vi "MM2KManCTRL.VI"(0 "MM System":u16(ring)=1 items=["MM3000", "MM2000"]) -> ()   [LabVIEW 2022 SP3]
uses:
  -MotionRoutines/MotionGlobals.vi
panel:
  in  "ExitSendCmd":bool
  out "Ax3Disp":dbl format="%.3f"
  out "Ax2Disp":dbl format="%.3f"
  in  "FineMi3":bool
  in  "FinePl3":bool
  in  "FineMi2":bool
  in  "FinePl2":bool
  in  "FineMi1":bool
  in  "FinePl1":bool
  in  "Rst3":bool
  in  "Ax3Plus":bool
  in  "Ax3Minus":bool
  in  "Rst2":bool
  in  "Ax2Plus":bool
  in  "Ax2Minus":bool
  in  "Rst1":bool
  out "Ax1Disp":dbl format="%.3f"
  in  "Ax1Plus":bool
  in  "Ax1Minus":bool
  # "Units are in cm.\n\"Rst\" zeros the position.\nBlue circles move 1 cm."
  # "X Axis"
  # "Y Axis"
  # "Z Axis"
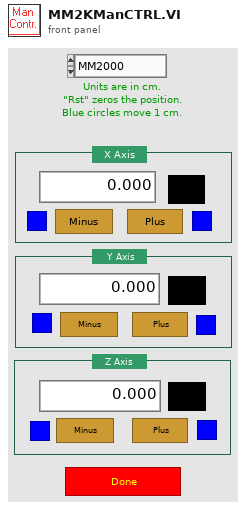
[diagram p1: front panel]
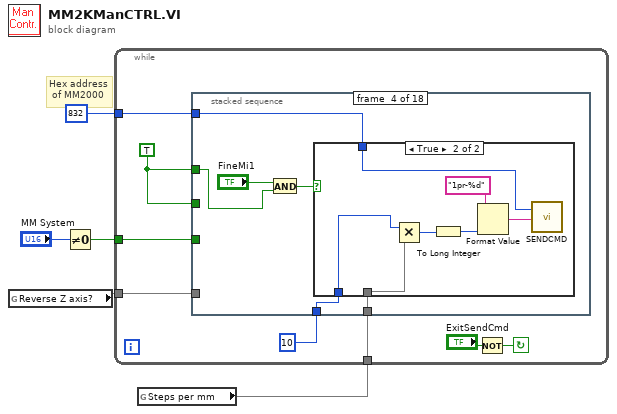
[diagram p0: block diagram]
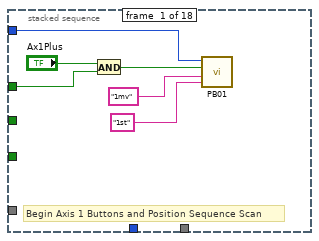
[diagram p2: hidden frame]
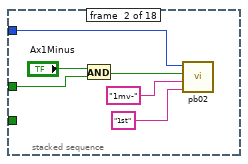
[diagram p3: hidden frame]
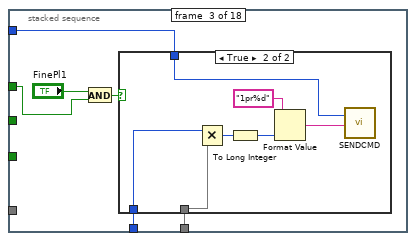
[diagram p4: hidden frame]
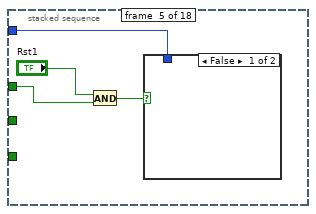
[diagram p7: hidden frame]
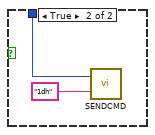
[diagram p8: hidden frame]
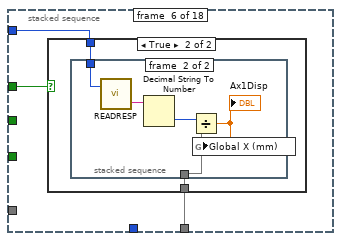
[diagram p9: hidden frame]
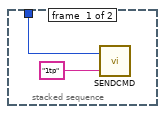
[diagram p11: hidden frame]
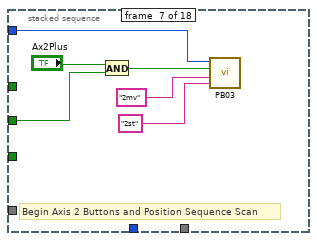
[diagram p12: hidden frame]
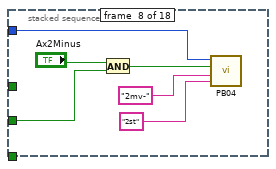
[diagram p13: hidden frame]
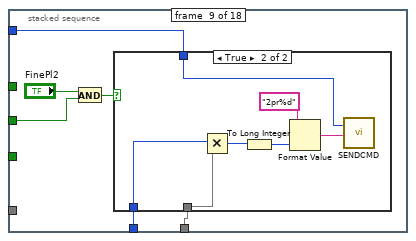
[diagram p14: hidden frame]
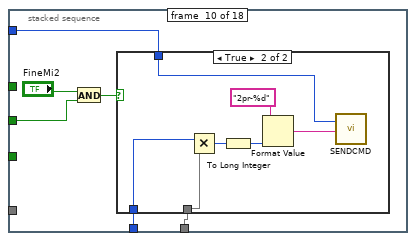
[diagram p16: hidden frame]
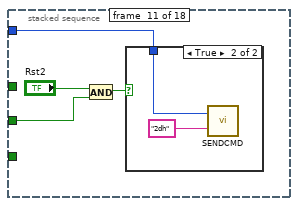
[diagram p18: hidden frame]
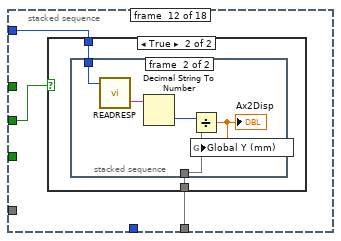
[diagram p20: hidden frame]
diagram:
  # "Hex address\n of MM2000"
  n1 = global read "MotionGlobals.vi" "Reverse Z axis?"() -> (w4)
  n2 = Not Equal To 0?(x="MM System") -> (x != 0?=w1:bool)
  n3 = global read "MotionGlobals.vi" "Steps per mm"() -> (w3)
  n4 = while {
    tunnel: w4 -> [w8]
    tunnel: w3 -> [w10]
    tunnel: u32 832 ("MotionMaster 2000 PC BUS Address") -> [w13]
    tunnel: w1 -> [w6]
    stop <- w11 continue-if-true
    w7 = TRUE
    n5 = stacked-sequence {
      tunnel: w7 -> [w16 w21 w28 w41 w53 w60 _ _ _ _ _ _ _ _ _ _ _ _]
      tunnel: w7 -> [_ _ _ _ _ _ w71 w77 w86 w99 w109 w115 _ _ _ _ _ _]
      tunnel: w6 -> [_ _ _ _ _ _ _ _ _ _ _ _ w131 w140 w147 w164 w179 w186]
      tunnel: w13 -> [w14 w20 w29 w42 w52 w59 w70 w76 w84 w97 w108 w116 w130 w139 w149 w166 w178 w187]
      tunnel: w10 -> [_ _ w27 w40 _ w58 _ _ w83 w96 _ w114 _ _ w146 w163 _ w185]
      tunnel: 10 -> [_ _ w26 w39 _ _ _ _ w82 w95 _ _ _ _ w145 w162 _ _]
      tunnel: w8 -> [_ _ _ _ _ _ _ _ _ _ _ _ w126 w135 w144 w161 _ w184]
      frame #0 {
        # "Begin Axis 1 Buttons and Position Sequence Scan"
        n6 = And(x="Ax1Plus", y=w16) -> (x .and. y?=w15:bool)
        n7 = call "PB01.VI"("Release Cmd"="1st", "Press Cmd"="1mv", "Button"=w15, "MM2000 Address"=w14) -> ()
      }
      frame #1 {
        n8 = And(x="Ax1Minus", y=w21) -> (x .and. y?=w23:bool)
        n9 = call "pb02.vi"("Release Cmd"="1st", "Press Cmd"="1mv-", "Button"=w23, "MM2000 Address"=w20) -> ()
      }
      frame #2 {
        n10 = And(x="FinePl1", y=w28) -> (x .and. y?=w31:bool)
        n11 = case shown="True" w31 {
          tunnel: w29 -> [_ w36]
          tunnel: w27 -> [_ w33]
          tunnel: w26 -> [_ w32]
          frame False {
          }
          frame True {
            n12 = Multiply(x=w32, y=w33) -> (x*y=w35:i32)
            n13 = To Long Integer(number=w35) -> (32bit integer=w34:i32)
            n14 = Format Value(format string="1pr%d", value (0)=w34) -> (output string=w38:string)  [unwired: 1 out]
            n15 = call "SENDCMD.VI"("MM2000 Command (ASCII String)"=w38, "MM2000 Address (Hexadecimal)"=w36) -> ()  [unwired: 1 in, 1 out]
          }
        }
      }
      frame #3 {
        n16 = And(x="FineMi1", y=w41) -> (x .and. y?=w44:bool)
        n17 = case shown="True" w44 {
          tunnel: w42 -> [_ w49]
          tunnel: w40 -> [_ w46]
          tunnel: w39 -> [_ w45]
          frame False {
          }
          frame True {
            n18 = Multiply(x=w45, y=w46) -> (x*y=w48:i32)
            n19 = To Long Integer(number=w48) -> (32bit integer=w47:i32)
            n20 = Format Value(format string="1pr-%d", value (0)=w47) -> (output string=w50:string)  [unwired: 1 out]
            n21 = call "SENDCMD.VI"("MM2000 Command (ASCII String)"=w50, "MM2000 Address (Hexadecimal)"=w49) -> ()  [unwired: 1 in, 1 out]
          }
        }
      }
      frame #4 {
        n22 = And(x="Rst1", y=w53) -> (x .and. y?=w55:bool)
        n23 = case shown="False" w55 {
          tunnel: w52 -> [_ w56]
          frame False {
          }
          frame True {
            n24 = call "SENDCMD.VI"("MM2000 Command (ASCII String)"="1dh", "MM2000 Address (Hexadecimal)"=w56) -> ()  [unwired: 1 in, 1 out]
          }
        }
      }
      frame #5 {
        n25 = case shown="True" w60 {
          tunnel: w59 -> [_ w62]
          tunnel: w58 -> [_ w61]
          frame False {
          }
          frame True {
            n26 = stacked-sequence {
              tunnel: w62 -> [w64 w69]
              tunnel: w61 -> [_ w65]
              frame #0 {
                n27 = call "SENDCMD.VI"("MM2000 Command (ASCII String)"="1tp", "MM2000 Address (Hexadecimal)"=w64) -> ()  [unwired: 1 in, 1 out]
              }
              frame #1 {
                n28 = call "READRESP.VI"("MM2000 Address (Hexadecimal)"=w69) -> ("MM2000 Response (ASCII String)"=w68:string)
                n29 = Decimal String To Number(string=w68) -> (number=w67:i32)  [unwired: 3 out]
                n30 = Divide(x=w67, y=w65) -> (x/y=w66:dbl)
                "Ax1Disp" <- w66
                n31 = global write "MotionGlobals.vi" "Global X (mm)"(w66) -> ()
              }
            }
          }
        }
      }
      frame #6 {
        # "Begin Axis 2 Buttons and Position Sequence Scan"
        n32 = And(x="Ax2Plus", y=w71) -> (x .and. y?=w73:bool)
        n33 = call "PB03.VI"("Release Cmd"="2st", "Press Cmd"="2mv", "Button"=w73, "MM2000 Address"=w70) -> ()
      }
      frame #7 {
        n34 = And(x="Ax2Minus", y=w77) -> (x .and. y?=w79:bool)
        n35 = call "PB04.VI"("Release Cmd"="2st", "Press Cmd"="2mv-", "Button"=w79, "MM2000 Address"=w76) -> ()
      }
      frame #8 {
        n36 = And(x="FinePl2", y=w86) -> (x .and. y?=w87:bool)
        n37 = case shown="True" w87 {
          tunnel: w84 -> [_ w92]
          tunnel: w83 -> [_ w89]
          tunnel: w82 -> [_ w88]
          frame False {
          }
          frame True {
            n38 = Multiply(x=w88, y=w89) -> (x*y=w91:i32)
            n39 = To Long Integer(number=w91) -> (32bit integer=w90:i32)
            n40 = Format Value(format string="2pr%d", value (0)=w90) -> (output string=w93:string)  [unwired: 1 out]
            n41 = call "SENDCMD.VI"("MM2000 Command (ASCII String)"=w93, "MM2000 Address (Hexadecimal)"=w92) -> ()  [unwired: 1 in, 1 out]
          }
        }
      }
      frame #9 {
        n42 = And(x="FineMi2", y=w99) -> (x .and. y?=w100:bool)
        n43 = case shown="True" w100 {
          tunnel: w97 -> [_ w105]
          tunnel: w96 -> [_ w102]
          tunnel: w95 -> [_ w101]
          frame False {
          }
          frame True {
            n44 = Multiply(x=w101, y=w102) -> (x*y=w104:i32)
            n45 = To Long Integer(number=w104) -> (32bit integer=w103:i32)
            n46 = Format Value(format string="2pr-%d", value (0)=w103) -> (output string=w106:string)  [unwired: 1 out]
            n47 = call "SENDCMD.VI"("MM2000 Command (ASCII String)"=w106, "MM2000 Address (Hexadecimal)"=w105) -> ()  [unwired: 1 in, 1 out]
          }
        }
      }
      frame #10 {
        n48 = And(x="Rst2", y=w109) -> (x .and. y?=w111:bool)
        n49 = case shown="True" w111 {
          tunnel: w108 -> [_ w112]
          frame False {
          }
          frame True {
            n50 = call "SENDCMD.VI"("MM2000 Command (ASCII String)"="2dh", "MM2000 Address (Hexadecimal)"=w112) -> ()  [unwired: 1 in, 1 out]
          }
        }
      }
      frame #11 {
        n51 = case shown="True" w115 {
          tunnel: w116 -> [_ w118]
          tunnel: w114 -> [_ w117]
          frame False {
          }
          frame True {
            n52 = stacked-sequence {
              tunnel: w118 -> [w119 w123]
              tunnel: w117 -> [_ w121]
              frame #0 {
                n53 = call "SENDCMD.VI"("MM2000 Command (ASCII String)"="2tp", "MM2000 Address (Hexadecimal)"=w119) -> ()  [unwired: 1 in, 1 out]
              }
              frame #1 {
                n54 = call "READRESP.VI"("MM2000 Address (Hexadecimal)"=w123) -> ("MM2000 Response (ASCII String)"=w125:string)
                n55 = Decimal String To Number(string=w125) -> (number=w124:i32)  [unwired: 3 out]
                n56 = Divide(x=w124, y=w121) -> (x/y=w122:dbl)
                "Ax2Disp" <- w122
                n57 = global write "MotionGlobals.vi" "Global Y (mm)"(w122) -> ()
              }
            }
          }
        }
      }
      frame #12 {
        # "Begin Axis 3 Buttons and Position Sequence Scan"
        n58 = And(x="Ax3Plus", y=w131) -> (x .and. y?=w133:bool)
        n59 = Select(t="3mv-", s=w126, f="3mv") -> (s? t:f=w127:string)
        n60 = call "PB05.VI"("Release Cmd"="3st", "Press Cmd"=w127, "Button"=w133, "MM2000 Address"=w130) -> ()
      }
      frame #13 {
        n61 = And(x="Ax3Minus", y=w140) -> (x .and. y?=w142:bool)
        n62 = Select(t="3mv", s=w135, f="3mv-") -> (s? t:f=w137:string)
        n63 = call "PB06.VI"("Release Cmd"="3st", "Press Cmd"=w137, "Button"=w142, "MM2000 Address"=w139) -> ()
      }
      frame #14 {
        n64 = And(x="FinePl3", y=w147) -> (x .and. y?=w150:bool)
        n65 = case shown="True" w150 {
          tunnel: w149 -> [_ w159]
          tunnel: w146 -> [_ w156]
          tunnel: w145 -> [_ w155]
          tunnel: w144 -> [_ w153]
          frame False {
          }
          frame True {
            n66 = Multiply(x=w155, y=w156) -> (x*y=w158:i32)
            n67 = Select(t="3pr-%d", s=w153, f="3pr%d") -> (s? t:f=w151:string)
            n68 = To Long Integer(number=w158) -> (32bit integer=w157:i32)
            n69 = Format Value(format string=w151, value (0)=w157) -> (output string=w160:string)  [unwired: 1 out]
            n70 = call "SENDCMD.VI"("MM2000 Command (ASCII String)"=w160, "MM2000 Address (Hexadecimal)"=w159) -> ()  [unwired: 1 in, 1 out]
          }
        }
      }
      frame #15 {
        n71 = And(x="FineMi3", y=w164) -> (x .and. y?=w167:bool)
        n72 = case shown="True" w167 {
          tunnel: w166 -> [_ w176]
          tunnel: w163 -> [_ w173]
          tunnel: w162 -> [_ w172]
          tunnel: w161 -> [_ w170]
          frame False {
          }
          frame True {
            n73 = Multiply(x=w172, y=w173) -> (x*y=w175:i32)
            n74 = Select(t="3pr%d", s=w170, f="3pr-%d") -> (s? t:f=w169:string)
            n75 = To Long Integer(number=w175) -> (32bit integer=w174:i32)
            n76 = Format Value(format string=w169, value (0)=w174) -> (output string=w177:string)  [unwired: 1 out]
            n77 = call "SENDCMD.VI"("MM2000 Command (ASCII String)"=w177, "MM2000 Address (Hexadecimal)"=w176) -> ()  [unwired: 1 in, 1 out]
          }
        }
      }
      frame #16 {
        n78 = And(x="Rst3", y=w179) -> (x .and. y?=w181:bool)
        n79 = case shown="True" w181 {
          tunnel: w178 -> [_ w182]
          frame False {
          }
          frame True {
            n80 = call "SENDCMD.VI"("MM2000 Command (ASCII String)"="3dh", "MM2000 Address (Hexadecimal)"=w182) -> ()  [unwired: 1 in, 1 out]
          }
        }
      }
      frame #17 {
        n81 = case shown="True" w186 {
          tunnel: w187 -> [_ w190]
          tunnel: w185 -> [_ w189]
          tunnel: w184 -> [_ w188]
          frame False {
          }
          frame True {
            n82 = stacked-sequence {
              tunnel: w190 -> [w191 w198]
              tunnel: w189 -> [_ w197]
              tunnel: w188 -> [_ w195]
              frame #0 {
                n83 = call "SENDCMD.VI"("MM2000 Command (ASCII String)"="3tp", "MM2000 Address (Hexadecimal)"=w191) -> ()  [unwired: 1 in, 1 out]
              }
              frame #1 {
                n84 = call "READRESP.VI"("MM2000 Address (Hexadecimal)"=w198) -> ("MM2000 Response (ASCII String)"=w200:string)
                n85 = Decimal String To Number(string=w200) -> (number=w199:i32)  [unwired: 3 out]
                n86 = Divide(x=w199, y=w197) -> (x/y=w194:dbl)
                n87 = Negate(x=w194) -> (-x=w193:dbl)
                n88 = Select(t=w193, s=w195, f=w194) -> (s? t:f=w196:dbl)
                "Ax3Disp" <- w196
                n89 = global write "MotionGlobals.vi" "Global  Z (mm)"(w196) -> ()
              }
            }
          }
        }
      }
    }
    n90 = Not(x="ExitSendCmd") -> (.not. x?=w11:bool)
  }
